vi "Frame_Size.vi"(8 "error in":errorcluster, 11 "camera handle in":u64) -> (0 "error out":errorcluster, 1 "Frame size (bytes)":i32, 3 "camera handle out":u64, 4 "Total pixel number":i32, 5 "PixelBitDepth (bits)":i32)   [LabVIEW 2014, in "PICam.lvlib"]
doc: "Reports the size, in bytes, of a data frame. If there was a single ROI definied, the frame size is equal with the ROI size in bytes!\n\n(X-pixels * Y-pixels * 2 byte; each pixel is represented on 2 Bytes monochrome values!)"
uses:
  PICam.lvlib
  Program Files/Princeton Instruments/PICam/Runtime/Picam32.dll
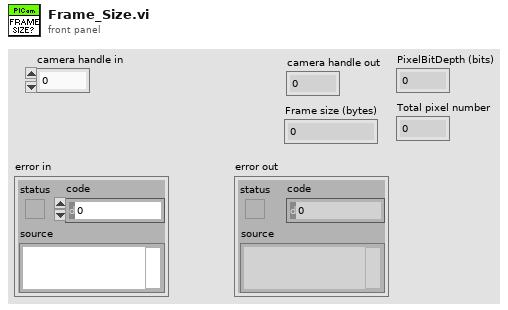
[diagram p1: front panel]
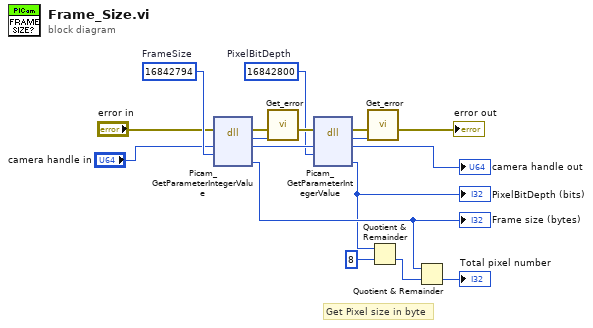
[diagram p0: block diagram]
diagram:
  w6 = u32 16842800  # PixelBitDepth
  w15 = u32 16842794  # FrameSize
  # "Get Pixel size in byte"
  n1 = dll-call lib="C:/Program Files/Princeton Instruments/PICam/Runtime/Picam32.dll" fn="Picam_GetParameterIntegerValue"(error in="error in", "camera"="camera handle in", "PicamParameter"=w15) -> (error out=w17:errorcluster, "return type"=w16:i32, "camera"=w7:u64, "FrameSize"=w12:i32)  [unwired: 4 in, 1 out]
  "Frame size (bytes)" <- w12
  n2 = call "Get_error.vi"("PICam_Error"=w16, "error in (no error)"=w17) -> ("error out"=w8:errorcluster)  [unwired: 9 in]
  n3 = dll-call lib="C:/Program Files/Princeton Instruments/PICam/Runtime/Picam32.dll" fn="Picam_GetParameterIntegerValue"(error in=w8, "camera"=w7, "PicamParameter"=w6) -> (error out=w9:errorcluster, "return type"=w10:i32, "camera"=→"camera handle out":u64, "PixelBitDepth"=w3:i32)  [unwired: 4 in, 1 out]
  "PixelBitDepth (bits)" <- w3
  n4 = call "Get_error.vi"("PICam_Error"=w10, "error in (no error)"=w9) -> ("error out"=→"error out":errorcluster)  [unwired: 9 in]
  n5 = Quotient & Remainder(x=w3, y=8) -> (floor(x/y)=w2:i32)  [unwired: 1 out]
  n6 = Quotient & Remainder(x=w12, y=w2) -> (floor(x/y)=→"Total pixel number":i32)  [unwired: 1 out]
